vi "Plugin.Transceiver Thread.Obtain.vi"(8 "error in (no error)":errorcluster, 11 "Plugin in":refnum<class "Plugin.lvclass">) -> (0 "error out":errorcluster, 2 "Transceiver Thread":refnum<class "Transceiver Interface.lvclass">, 3 "Plugin out":refnum<class "Plugin.lvclass">)   [LabVIEW 2017, in "DSF Core.lvlib" / "Plugin.lvclass"]
uses:
  Plugin.lvclass
  Interfaces/Transceiver Interface/Transceiver Interface.lvclass
  Plugin.lvclass/Plugin.ctl
  Thread Pool/Pool.lvclass/Pool.ctl
  Debug/FIFO Flags/FIFO Flags.lvclass/FIFO Flags.ctl
  Thread Pool/Read FIFO.vi
  Thread Pool/Get FIFO.vi
  Thread Pool/Get Debug Flags.vi
  Debug/FIFO Flags/Get Infinite Timeouts.vi
  Thread Pool/ID Pool.lvclass
  C:/github/data-sharing-framework/Data Sharing Framework/Source/Core/Engine/Classes/Thread Pool/Pool.lvclass
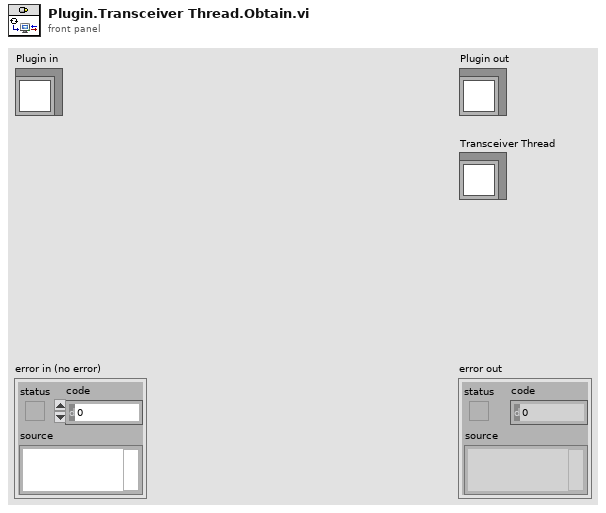
[diagram p1: front panel]
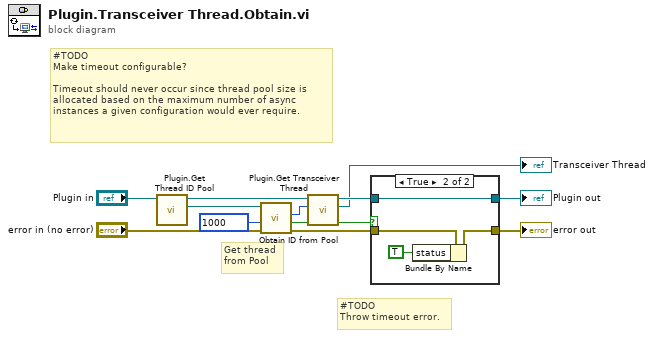
[diagram p0: block diagram]
diagram:
  # "#TODO\nThrow timeout error."
  # "#TODO\nMake timeout configurable?\n\nTimeout should never occur since thread pool size is allocated based on the maximum number of async instances a given configuration would ever require."
  # "Get thread from Pool"
  n1 = call "Plugin.Get Thread ID Pool.vi"("Plugin in"="Plugin in") -> ("Thread ID Pool"=w10:refnum<class "ID Pool.lvclass">, "Plugin out"=w8:refnum<class "Plugin.lvclass">)  [unwired: 9 in]
  n2 = call "Obtain ID from Pool.vi"("error in (no error)"="error in (no error)", "timeout in ms (0)"=1000, "ID Pool in"=w10) -> ("error out"=w6:errorcluster, "timed out?"=w4:bool, "id"=w7:i32)  [unwired: 5 in, 1 out]
  n3 = call "Plugin.Get Transceiver Thread.vi"("index"=w7, "Plugin in"=w8) -> ("Transceiver Thread"=→"Transceiver Thread":refnum<class "Transceiver Interface.lvclass">, "Plugin out"=w3:refnum<class "Plugin.lvclass">)  [unwired: 8 in]
  n4 = case shown="True" w4 {
    tunnel: w6 -> [w14 w18]
    tunnel: [w14 w16] -> w5
    tunnel: w3 -> [w13 w15]
    tunnel: [w13 w15] -> w2
    frame False {
    }
    frame True {
      n5 = Bundle By Name(cluster=w18, "status"=TRUE) -> (w16:errorcluster)
    }
  }
  "error out" <- w5
  "Plugin out" <- w2
